vi "receive.vi"(0 "Subnet in":refnum<class "Subnet.lvclass">, 11 "error in (no error)":errorcluster) -> (4 "Subnet out":refnum<class "Subnet.lvclass">, 6 "ValidCRC":i32, 8 "InvalidCRC":i32, 10 "Messages":i32, 14 "CRCIssues":T1[](array[typedef]) {"Data" format="%02x"}, 15 "error out":errorcluster)   [LabVIEW 2016, in "Subnet.lvclass"]
uses:
  Subnet.lvclass
  Common_RT_Modbus/DataTypes/RxFrame.ctl
  Subnet.lvclass/Subnet.ctl
  Common_RT_Modbus/DynamicFrameParser/DynamicFrameParser.lvclass
  Common_RT_Modbus/IModbus/IModbus.lvclass
  Common_RT_HPILC/HPILC/HPILC.lvclass
  Common_RT_MTILC/MTILC/MTILC.lvclass
  Common_RT_MDILC/MDILC/MDILC.lvclass
  Common_RT_MIILC/MIILC/MIILC.lvclass
  Common_RT_Modbus/RTModbus.lvlib
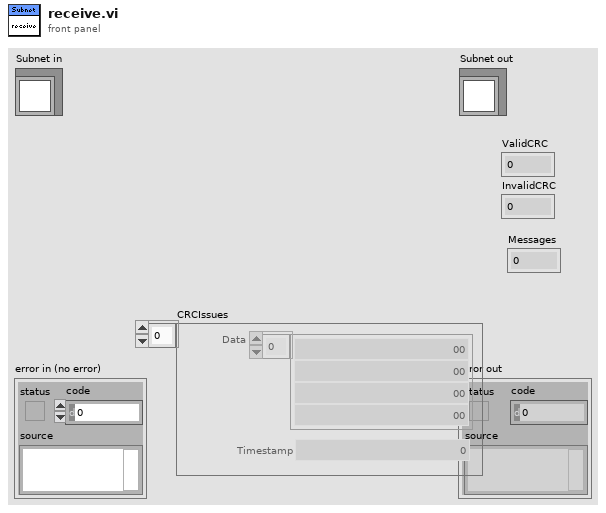
[diagram p1: front panel]
types:
  T1 = typedef "RTModbus.lvlib/RxFrame.ctl" = cluster{"Data":u8[], "Timestamp":u64}
  T2 = typedef "ILCIndexData.ctl" = cluster{"ILCTypes":T3, "Index":i32}
  T3 = typedef "ILCTypes.ctl" = enum16{"Undefined", "SAA", "DAA", "HP", "MT", "MD", "MI"}
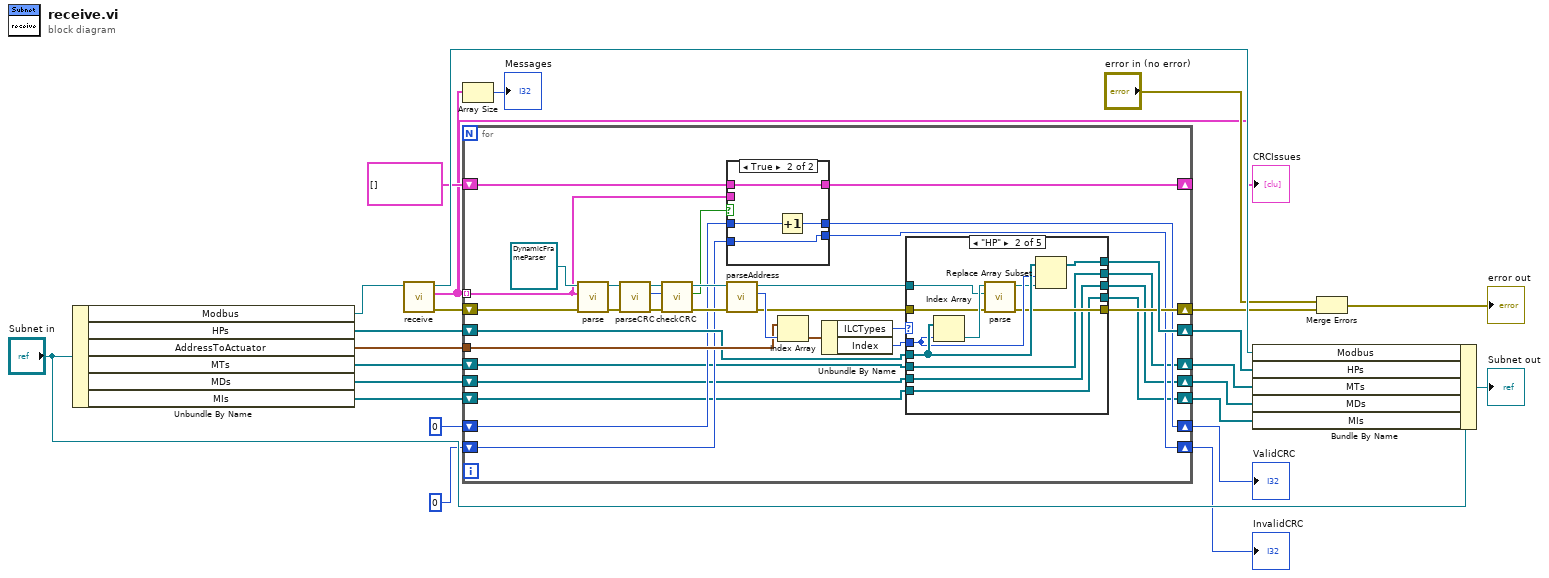
[diagram p0: block diagram]
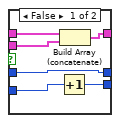
[diagram p2: hidden frame]
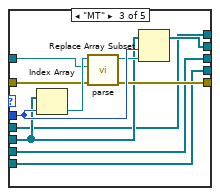
[diagram p4: hidden frame]
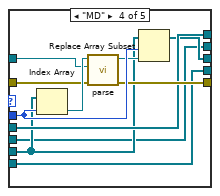
[diagram p5: hidden frame]
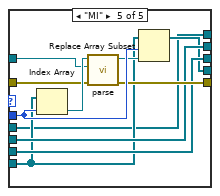
[diagram p6: hidden frame]
diagram:
  n1 = Unbundle By Name("Subnet in") -> ("Modbus"=w24:refnum<class "IModbus.lvclass">, "HPs"=w22:refnum<class "HPILC.lvclass">[], "AddressToActuator"=w23:T2[], "MTs"=w8:refnum<class "MTILC.lvclass">[], "MDs"=w6:refnum<class "MDILC.lvclass">[], "MIs"=w4:refnum<class "MIILC.lvclass">[])
  n2 = call-dynamic "receive.vi"("IModbus in"=w24) -> ("error out"=w17:errorcluster, "Data"=w1:T1[], "IModbus out"=w20:refnum<class "IModbus.lvclass">)  [unwired: 8 in]
  "CRCIssues" <- w1
  n3 = Array Size(array=w1) -> (size(s)=→"Messages":i32)
  n4 = for {
    tunnel: w1 -> [w27] mode=indexing
    tunnel: w23 -> [w55]
    shift-right: [w50] -> w19
    shift-left: w22 -> [w52]
    shift-right: [w46] -> w14
    shift-left: w17 -> [w48]
    shift-right: [w36] -> w11
    shift-left: 0 -> [w37]
    shift-right: [w35] -> w10
    shift-left: 0 -> [w34]
    shift-right: [w32] -> w7
    shift-left: w8 -> [w33]
    shift-right: [w30] -> w5
    shift-left: w6 -> [w31]
    shift-right: [w28] -> w3
    shift-left: w4 -> [w29]
    shift-right: [w26] -> _
    shift-left: T1[] [] -> [w25]
    n5 = call "parse.vi"("error in (no error)"=w48, "RxFrame"=w27, "FrameParser in"=refnum<class "DynamicFrameParser.lvclass"> refnum ("RTModbus.lvlib:DynamicFrameParser.lvclass")) -> ("error out"=w44:errorcluster, "FrameParser out"=w40:refnum<class "DynamicFrameParser.lvclass">)  [unwired: 7 in]
    n6 = call "parseCRC.vi"("error in (no error)"=w44, "FrameParser in"=w40) -> ("error out"=w43:errorcluster, "CRC"=w45:u16, "FrameParser out"=w39:refnum<class "DynamicFrameParser.lvclass">)  [unwired: 7 in]
    n7 = call "checkCRC.vi"("error in (no error)"=w43, "CRC"=w45, "FrameParser in"=w39) -> ("error out"=w42:errorcluster, "Valid"=w38:bool, "FrameParser out"=w41:refnum<class "DynamicFrameParser.lvclass">)  [unwired: 6 in]
    n8 = case shown="True" w38 {
      tunnel: w37 -> [w61 w67]
      tunnel: [w61 w66] -> w36
      tunnel: [w62 w65] -> w35
      tunnel: w34 -> [w63 w65]
      tunnel: w27 -> [w60 _]
      tunnel: [w59 w64] -> w26
      tunnel: w25 -> [w58 w64]
      frame False {
        n9 = Increment(x=w63) -> (x+1=w62:i32)
        n10 = Build Array (concatenate)(w58, w60) -> (w59:T1[])
      }
      frame True {
        n11 = Increment(x=w67) -> (x+1=w66:i32)
      }
    }
    n12 = call "parseAddress.vi"("error in (no error)"=w42, "FrameParser in"=w41) -> ("error out"=w47:errorcluster, "Address"=w56:u8, "FrameParser out"=w49:refnum<class "DynamicFrameParser.lvclass">)  [unwired: 7 in]
    n13 = Index Array(array=w55, index=w56) -> (element=w54:T2)
    n14 = Unbundle By Name(w54) -> ("ILCTypes"=w53:T3, "Index"=w51:i32)
    n15 = case shown="\"HP\"" w53 {
      tunnel: w52 -> [w72 w83 w86 w99 w106]
      tunnel: w51 -> [_ w81 w94 w105 w116]
      tunnel: [w72 w82 w86 w99 w106] -> w50
      tunnel: w49 -> [_ w78 w91 w102 w113]
      tunnel: w47 -> [w71 w77 w90 w101 w112]
      tunnel: [w71 w76 w89 w100 w111] -> w46
      tunnel: w33 -> [w70 w75 w88 w96 w110]
      tunnel: [w70 w75 w87 w96 w110] -> w32
      tunnel: w31 -> [w69 w74 w85 w98 w109]
      tunnel: [w69 w74 w85 w97 w109] -> w30
      tunnel: [w68 w73 w84 w95 w107] -> w28
      tunnel: w29 -> [w68 w73 w84 w95 w108]
      frame "Undefined", Default {
      }
      frame "HP" {
        n16 = Index Array(array=w83, index=w81) -> (element=w79:refnum<class "HPILC.lvclass">)
        n17 = call-dynamic "parse.vi"("error in (no error)"=w77, "DynamicFrameParser"=w78, "HPILC in"=w79) -> ("error out"=w76:errorcluster, "HPILC out"=w80:refnum<class "HPILC.lvclass">)  [unwired: 6 in, 1 out]
        n18 = Replace Array Subset(array=w83, new element=w80, index=w81) -> (w82:refnum<class "HPILC.lvclass">[])
      }
      frame "MT" {
        n19 = Index Array(array=w88, index=w94) -> (element=w92:refnum<class "MTILC.lvclass">)
        n20 = call-dynamic "parse.vi"("error in (no error)"=w90, "DynamicFrameParser"=w91, "MTILC in"=w92) -> ("error out"=w89:errorcluster, "MTILC out"=w93:refnum<class "MTILC.lvclass">)  [unwired: 6 in, 1 out]
        n21 = Replace Array Subset(array=w88, new element=w93, index=w94) -> (w87:refnum<class "MTILC.lvclass">[])
      }
      frame "MD" {
        n22 = Index Array(array=w98, index=w105) -> (element=w103:refnum<class "MDILC.lvclass">)
        n23 = call-dynamic "parse.vi"("error in (no error)"=w101, "DynamicFrameParser"=w102, "MDILC in"=w103) -> ("error out"=w100:errorcluster, "MDILC out"=w104:refnum<class "MDILC.lvclass">)  [unwired: 6 in, 1 out]
        n24 = Replace Array Subset(array=w98, new element=w104, index=w105) -> (w97:refnum<class "MDILC.lvclass">[])
      }
      frame "MI" {
        n25 = Index Array(array=w108, index=w116) -> (element=w114:refnum<class "MIILC.lvclass">)
        n26 = call-dynamic "parse.vi"("error in (no error)"=w112, "DynamicFrameParser"=w113, "MIILC in"=w114) -> ("error out"=w111:errorcluster, "MIILC out"=w115:refnum<class "MIILC.lvclass">)  [unwired: 6 in, 1 out]
        n27 = Replace Array Subset(array=w108, new element=w115, index=w116) -> (w107:refnum<class "MIILC.lvclass">[])
      }
    }
  }
  "ValidCRC" <- w11
  "InvalidCRC" <- w10
  n28 = Bundle By Name(cluster="Subnet in", "Modbus"=w20, "HPs"=w19, "MTs"=w7, "MDs"=w5, "MIs"=w3) -> (→"Subnet out":refnum<class "Subnet.lvclass">)
  n29 = Merge Errors("error in (no error)", w14) -> (→"error out":errorcluster)
